vi "fgv_DL950_q.vi"(7 "cmd":T2, 8 "error in":errorcluster, 11 "data":T1=enum."start") -> (0 "error out":errorcluster, 3 "queue out":refnum<queue>)   [LabVIEW 2019]
uses:
  _ctrl/create-rw-close.ctl
  _ctrl/start.ctl
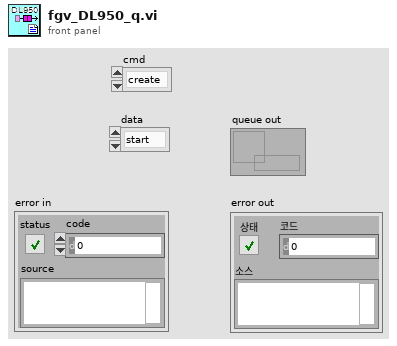
[diagram p1: front panel]
types:
  T1 = typedef "start.ctl" = enum16{"init", "open", "set", "start", "stop", "read", "read_items", "query", "close", "T_single", "reset", "exit"}
  T2 = typedef "create-rw-close.ctl" = enum16{"create", "write", "read", "delete", "close"}
  T3 = typedef "system-status_내구.ctl" = enum16{"Initial", "Update", "Clear"}
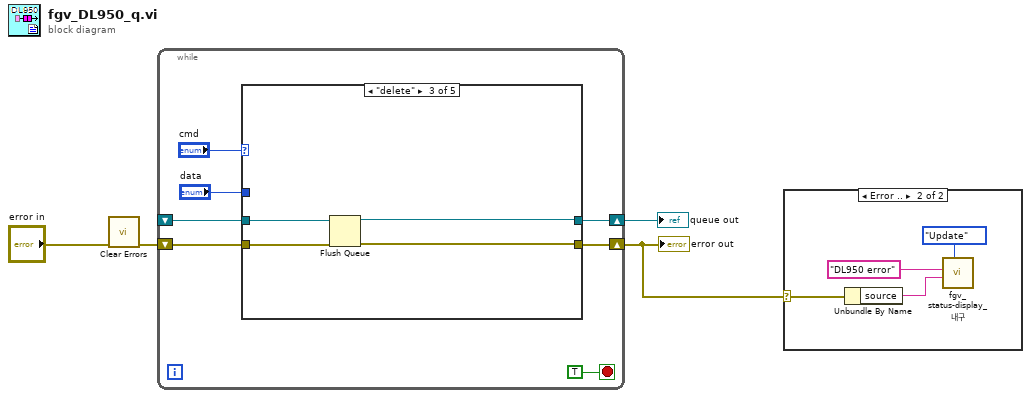
[diagram p0: block diagram]
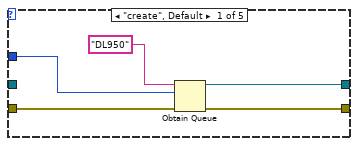
[diagram p3: hidden frame]
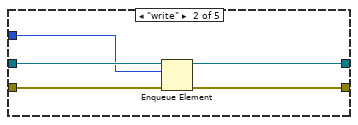
[diagram p4: hidden frame]
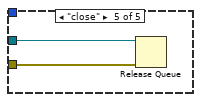
[diagram p6: hidden frame]
diagram:
  n1 = call <vilib>:"Clear Errors.vi"("error in (no error)"="error in") -> ("error out"=w2:errorcluster)  [unwired: 5 in, 1 out]
  n2 = while {
    shift-right: [w8] -> w4
    shift-left: _ -> [w5]
    shift-right: [w7] -> w1
    shift-left: w2 -> [w9]
    stop <- TRUE stop-if-true
    n3 = case shown="\"delete\"" "cmd" {
      tunnel: w9 -> [w16 w20 w23 w26 w29]
      tunnel: [w15 w19 w24 w27 _] -> w8
      tunnel: [w14 w18 w22 w26 _] -> w7
      tunnel: "data" -> [w12 w17 _ _ _]
      tunnel: w5 -> [_ w21 w25 w27 w28]
      frame "create", Default {
        n4 = Obtain Queue(name (unnamed)="DL950" ("이름(이름없음)"), element data type=w12, error in (no error)=w16) -> (queue out=w15:refnum<queue>, error out=w14:errorcluster)  [unwired: 2 in, 1 out]
      }
      frame "write" {
        n5 = Enqueue Element(queue=w21, element=w17, error in (no error)=w20) -> (queue out=w19:refnum<queue>, error out=w18:errorcluster)  [unwired: 1 in, 1 out]
      }
      frame "delete" {
        n6 = Flush Queue(queue=w25, error in (no error)=w23) -> (queue out=w24:refnum<queue>, error out=w22:errorcluster)  [unwired: 1 out]
      }
      frame "read" {
      }
      frame "close" {
        n7 = Release Queue(queue=w28, error in (no error)=w29) -> ()  [unwired: 1 in, 3 out]
      }
    }
  }
  "queue out" <- w4
  "error out" <- w1
  n8 = case shown="Error .." w1 {
    selector: w1 -> [_ w31]
    frame No Error {
    }
    frame Error {
      n9 = Unbundle By Name(w31) -> ("source"=w30:string)
      n10 = call "fgv_status-display_내구.vi"("Mode"=system-status_내구."Update", "detail"=w30, "title"="DL950 error") -> ()  [unwired: 8 in, 1 out]
    }
  }
